vi "Gather State Data.vi"(8 "error in (no error)":errorcluster) -> (0 "error out":errorcluster)   [LabVIEW 2015, in "State Accessor Scripter.lvclass"]
uses:
  State Accessor Scripter.lvclass
panel:
  out "Variant":variant
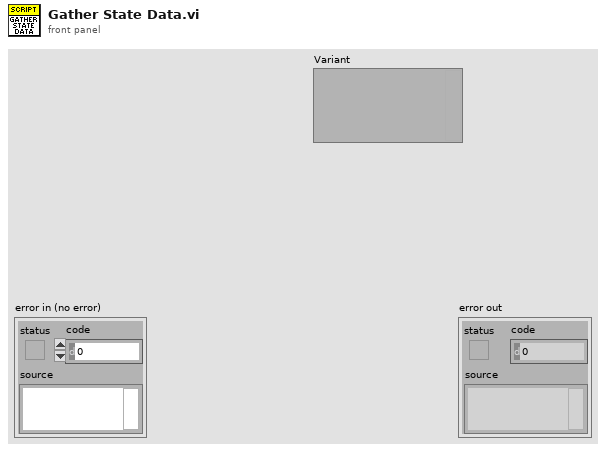
[diagram p1: front panel]
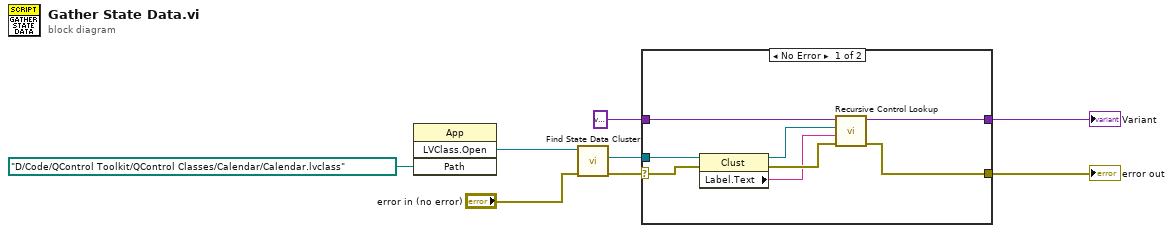
[diagram p0: block diagram]
diagram:
  n1 = invoke class="App" method="LVClass.Open"("Path"=path "D:/Code/QControl Toolkit/QControl Classes/Calendar/Calendar.lvclass") -> ("LVClass.Open"=w8:refnum<vi>)  [unwired: 3 in, 3 out]
  n2 = call "Find State Data Cluster.vi"("error in (no error)"="error in (no error)", "QControl Class Refnum in"=w8) -> ("error out"=w4:errorcluster, "State Data Cluster"=w6:refnum<vi>)  [unwired: 7 in, 1 out]
  n3 = case shown="No Error" w4 {
    selector: w4 -> [w14 w18]
    tunnel: w6 -> [w16 _]
    tunnel: variant -> [w12 w17]
    tunnel: [w10 w18] -> w2
    tunnel: [w9 w17] -> w1
    frame No Error {
      n4 = property class="Clust"(reference=w16, error in=w14) -> (reference out=w11:refnum<vi>, error out=w15:errorcluster, "Label.Text"=w13:string)
      n5 = call "Recursive Control Lookup.vi"("error in (no error)"=w15, "Tag"=w13, "Cluster in"=w11, "Lookup Table in"=w12) -> ("error out"=w10:errorcluster, "Lookup Table in"=w9:variant)  [unwired: 6 in]
    }
    frame Error {
    }
  }
  "error out" <- w2
  "Variant" <- w1
